vi "1D sweep step calculator (SubVI).vi"(6 "Iteration":dbl, 9 "Number of steps":dbl, 10 "Minimum current":dbl, 11 "Maximum current":dbl) -> (3 "Current at this iteration":dbl)   [LabVIEW 2018]
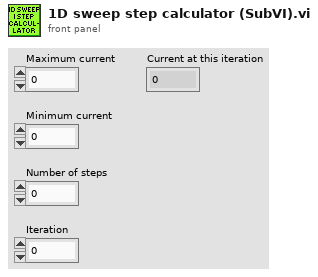
[diagram p1: front panel]
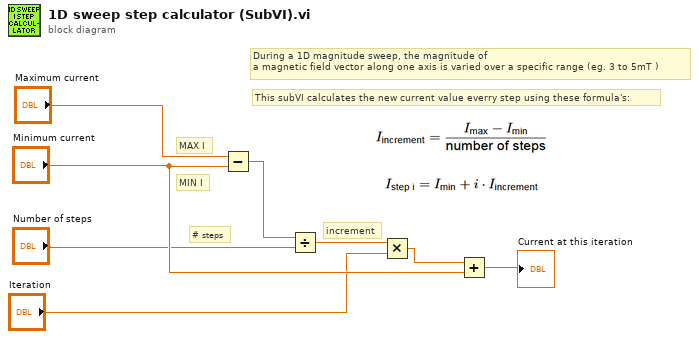
[diagram p0: block diagram]
diagram:
  # "This subVI calculates the new current value everry step using these formula's:"
  # "During a 1D magnitude sweep, the magnitude of\na magnetic field vector along one axis is varied over a specific range (eg. 3 to 5mT )"
  # "increment"
  # "# steps"
  # "MIN I"
  # "MAX I"
  n1 = Subtract(x="Maximum current", y="Minimum current") -> (x-y=w2:dbl)
  n2 = Divide(x=w2, y="Number of steps") -> (x/y=w4:dbl)
  n3 = Multiply(x=w4, y="Iteration") -> (x*y=w7:dbl)
  n4 = Add(x=w7, y="Minimum current") -> (x+y=→"Current at this iteration":dbl)
